vi "CTL Simulate Pump.vi"(6 "error in (no error)":errorcluster, 7 "Full Config":T1={"Bench Config"={"Name"="OLR001", {"Step Levels"=0.05, "Tolerance"=0.01, "Sample Rate"=0.05, "Resistor"=100.0, "M Level Cal"=1.0, "[B Level Cal"=0.0, "Max Fill Rate"=0.025, "Max Gal"=10.0, "Max Inches"=10.0}}, "Test Value Table "=[[0.0, 0.0, 0.0, 0.0, 0.0, 0.0, 0.0, 0.0, 0.0, 0.0], [100.0, 2.0, 7.91, 8.01, 7.55, 7.65, 7.685, 7.785, 7.325, 7.425], [200.0, 3.0, 7.46, 7.56, 7.1, 7.2, 7.235, 7.335, 6.875, 6.975], [300.0, 4.0, 7.01, 7.11, 6.65, 6.75, 6.785, 6.885, 6.425, 6.525], [400.0, 5.0, 6.56, 6.66, 6.2, 6.3, 6.335, 6.435, 5.975, 6.075], [500.0, 6.0, 6.11, 6.21, 5.75, 5.85, 5.885, 5.985, 5.525, 5.625], [600.0, 7.0, 5.66, 5.76, 5.3, 5.4, 5.435, 5.535, 5.075, 5.175], [700.0, 8.0, 5.21, 5.31, 4.85, 4.95, 4.985, 5.085, 4.625, 4.725], [800.0, 9.0, 4.76, 4.86, 4.4, 4.5, 4.535, 4.635, 4.175, 4.275], [900.0, 10.0, 4.31, 4.41, 3.95, 4.05, 4.085, 4.185, 3.725, 3.825], [1000.0, 11.0, 3.86, 3.96, 3.5, 3.6, 3.635, 3.735, 3.275, 3.375], [1100.0, 12.0, 3.41, 3.51, 3.05, 3.15, 3.185, 3.285, 2.825, 2.925]], "Table Col Titles"=[["A Resist", "A Tolerence", "A Fill Lo", "A Fill Hi", "A Drain Lo", "A Drain Hi", "B Fill Lo", "B Fill Hi", "B Drain Lo", "B Drain Hi"]], "Pump CtlRef In"={"Fill "=refnum, "Drain"=refnum, "Level PV"=refnum, "Flow Rate%"=refnum, "Run Test"=refnum, "Sim"=refnum, "Jog"=refnum}, "Bench Status"={"Pump Status"=refnum, "Instrumnet\n Status"=refnum}}, 9 "Level PV":dbl=0.024999999999999842, 10 "Level SP":dbl, 11 "TEST STATUS In":T5(ring)=enum."Done") -> (0 "error out":errorcluster, 1 "Level OUt":dbl=0.024999999999999842, 2 "Level Sense":dbl=0.014999999999999904, 3 "TEST STATUS Out":T5(ring)=enum."Done")   [LabVIEW 2024]
uses:
  Control Definitions/Def FullCfg.ctl
  Control Definitions/Def BenchCfg.ctl
  Control Definitions/Def PumpCtlRefs.ctl
  Control Definitions/Def Bench Status.ctl
panel:
  in  "Constant":dbl=8.5 format="%#_13g"
  in  "Slope":dbl=-0.6 format="%#_13g"
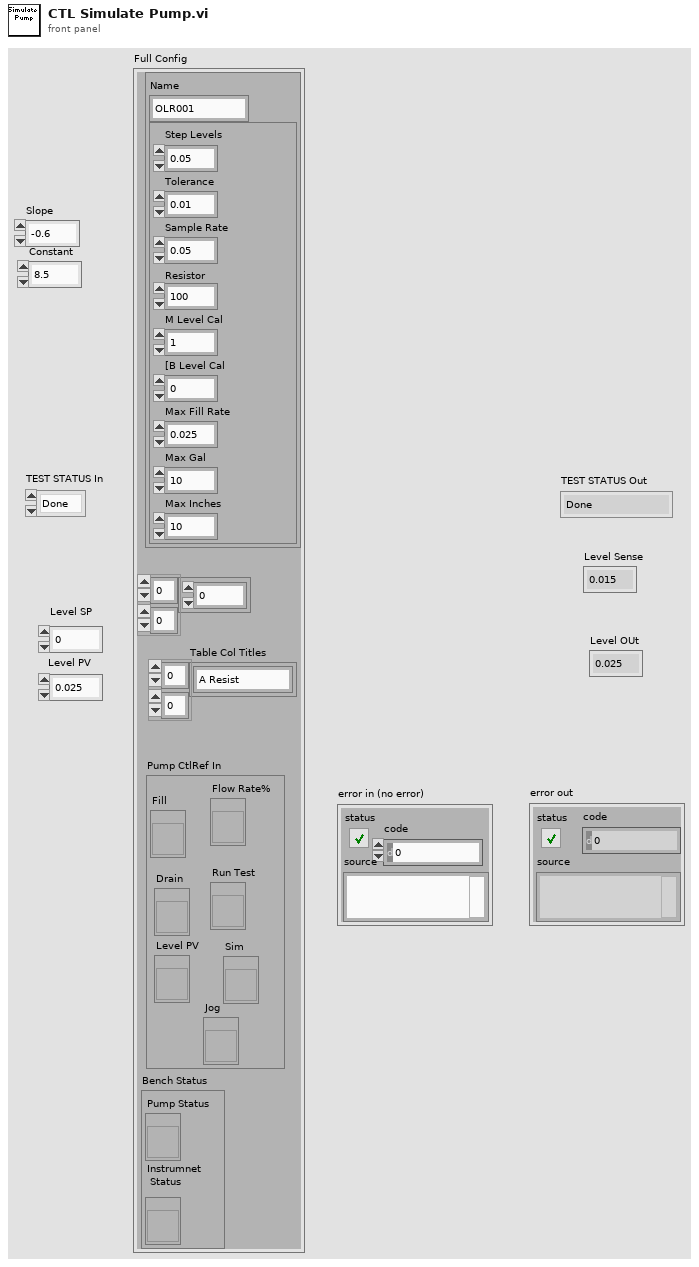
[diagram p1: front panel]
types:
  T1 = typedef "Def FullCfg.ctl" = cluster{"Bench Config":T2, "Test Value Table ":dbl[][], "Table Col Titles":string[][], "Pump CtlRef In":T3, "Bench Status":T4}
  T2 = typedef "Def BenchCfg.ctl" = cluster{"Name":string, cluster{"Step Levels":dbl, "Tolerance":dbl, "Sample Rate":dbl, "Resistor":dbl, "M Level Cal":dbl, "[B Level Cal":dbl, "Max Fill Rate":dbl, "Max Gal":dbl, "Max Inches":dbl}}
  T3 = typedef "Def PumpCtlRefs.ctl" = cluster{"Fill ":refnum<vi>, "Drain":refnum<vi>, "Level PV":refnum<vi>, "Flow Rate%":refnum<vi>, "Run Test":refnum<vi>, "Sim":refnum<vi>, "Jog":refnum<vi>}
  T4 = typedef "Def Bench Status.ctl" = cluster{"Pump Status":refnum<vi>, "Instrumnet\n Status":refnum<vi>}
  T5 = enum16{"MANUAL", "Start", "Filling", "FULL", "Draining", "EMPTY", "Done"}
  T6 = cluster{"Step Levels":dbl, "Tolerance":dbl, "Sample Rate":dbl, "Resistor":dbl, "M Level Cal":dbl, "[B Level Cal":dbl, "Max Fill Rate":dbl, "Max Gal":dbl, "Max Inches":dbl}
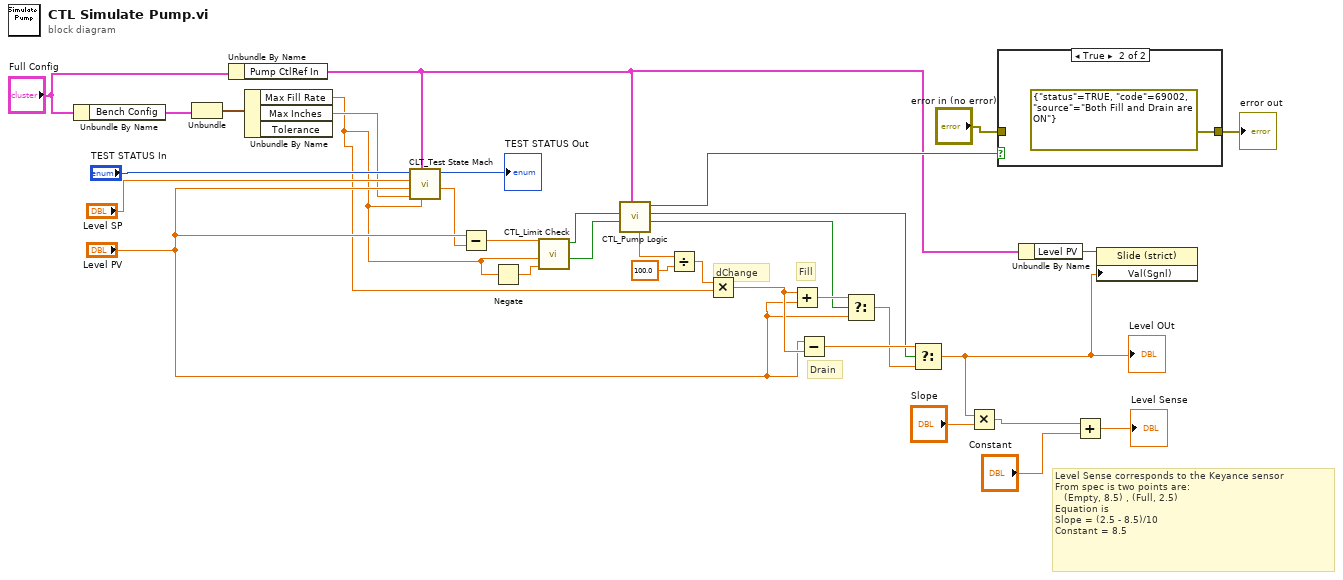
[diagram p0: block diagram]
diagram:
  # "Level Sense corresponds to the Keyance sensor\nFrom spec is two points are:\n   (Empty, 8.5) , (Full, 2.5)\nEquation is \nSlope = (2.5 - 8.5)/10\nConstant = 8.5"
  # "dChange"
  # "Drain"
  # "Fill"
  n1 = Unbundle By Name("Full Config") -> ("Bench Config"=w18:T2)
  n2 = Unbundle(w18) -> (w17:T6)  [unwired: 1 out]
  n3 = Unbundle By Name("Full Config") -> ("Pump CtlRef In"=w7:T3)
  n4 = Unbundle By Name(w17) -> ("Max Fill Rate"=w6:dbl, "Max Inches"=w16:dbl)  [unwired: 1 out]
  n5 = call "CLT_Test State Mach.vi"("Tolerance"=w6, "Pump CtlRef In"=w7, "Max Fill in"=w16, "Level PV"="Level PV", "Level SP"="Level SP", "TEST STATUS In"="TEST STATUS In") -> ("SP out"=w21:dbl, "TEST STATUS Out"=→"TEST STATUS Out":T5)  [unwired: 4 in]
  n6 = Subtract(x="Level PV", y=w21) -> (x-y=w25:dbl)
  n7 = Negate(x=w6) -> (-x=w24:dbl)
  n8 = call "CTL_Limit Check.vi"("Neg Limit"=w24, "Pos Limit"=w6, "X"=w25) -> ("X< Neg"=w14:bool, "X>Pos"=w15:bool)  [unwired: 6 in, 1 out]
  n9 = call "CTL_Pump Logic.vi"("Pump CtlRef In"=w7, "Fill Cmd"=w14, "Drain Cmd"=w15) -> ("Fill Out"=w12:bool, "Drain Out"=w11:bool, "Err"=w10:bool, "Flow Rate"=w13:dbl)  [unwired: 4 in, 1 out]
  n10 = Divide(x=w13, y=100.0) -> (x/y=w27:dbl)
  n11 = Multiply(x=w27, y=w6) -> (x*y=w26:dbl)
  n12 = Add(x=w26, y="Level PV") -> (x+y=w33:dbl)
  n13 = Subtract(x="Level PV", y=w26) -> (x-y=w32:dbl)
  n14 = Select(t=w33, s=w12, f="Level PV") -> (s? t:f=w31:dbl)
  n15 = Select(t=w32, s=w11, f=w31) -> (s? t:f=w5:dbl)
  "Level OUt" <- w5
  n16 = Multiply(x=w5, y="Slope") -> (x*y=w1:dbl)
  n17 = case shown="True" w10 {
    tunnel: "error in (no error)" -> [w34 _]
    tunnel: [w34 errorcluster {"status"=TRUE, "code"=69002, "source"="Both Fill and Drain are ON"} ("error in (no error)")] -> w29
    frame False {
    }
    frame True {
    }
  }
  "error out" <- w29
  n18 = Unbundle By Name(w7) -> ("Level PV"=w8:refnum<vi>)
  n19 = Add(x=w1, y="Constant") -> (x+y=→"Level Sense":dbl)
  n20 = property on="Property Node" class="Slide (strict)"(reference=w8, "Val(Sgnl)"=w5) -> ()  [unwired: 1 in, 2 out]
